vi "Grab Versions.vi"() -> (2 "Selection":string, 3 "Strings and Values":cluster{"string":string, "value":string}[](array[cluster]))   [LabVIEW 2021, in "TSC Button Editor.lvclass"]
doc: "See all of the available versions to save the button for compatiblity.\n\n<b>Code Developed By:</b>\nTechnology Service Corporation\n1983 S Liberty Drive\nBloomington, IN 47403\nwww.tsc.com/atcs\n\nDeveloper:\nDaniel Coons"
uses:
  TSC Button Editor.lvclass
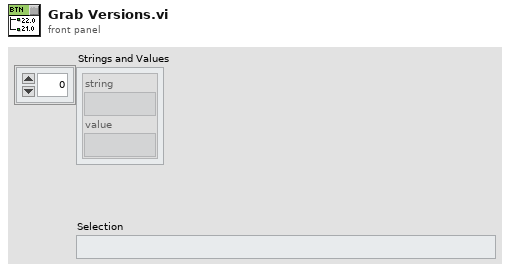
[diagram p1: front panel]
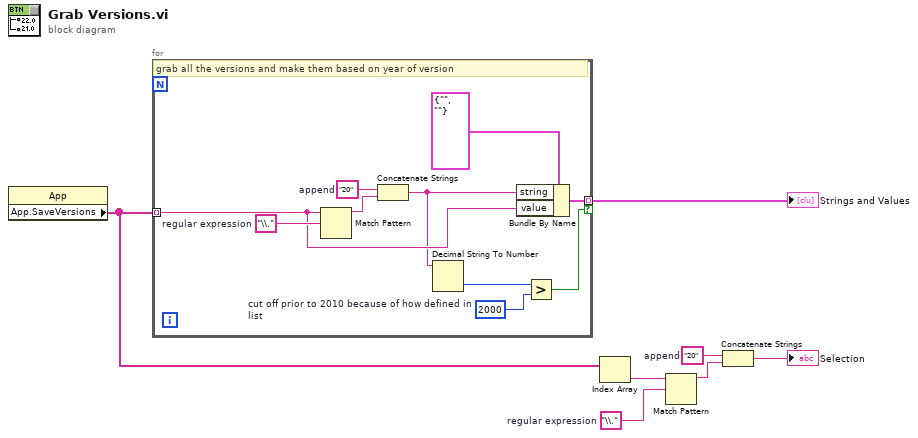
[diagram p0: block diagram]
diagram:
  w3 = "20"  # append
  w5 = "\\."  # regular expression
  n1 = property class="App"() -> ("App.SaveVersions"=w2:string[])  [unwired: 2 in, 2 out]
  n2 = for {
    tunnel: w2 -> [w13] mode=indexing
    tunnel: [w12] -> w1 mode=indexing if=w8
    w9 = 2000  # cut off prior to 2010 because of how defined in list
    w15 = "20"  # append
    w17 = "\\."  # regular expression
    # "grab all the versions and make them based on year of version"
    n3 = Match Pattern(string=w13, regular expression=w17) -> (before substring=w16:string)  [unwired: 1 in, 3 out]
    n4 = Concatenate Strings(w15, w16) -> (w11:string)
    n5 = Decimal String To Number(string=w11) -> (number=w10:i32)  [unwired: 2 in, 1 out]
    n6 = Bundle By Name(cluster=cluster{"string":string, "value":string} {"string"="", "value"=""}, "string"=w11, "value"=w13) -> (w12:cluster{"string":string, "value":string})
    n7 = Greater?(x=w10, y=w9) -> (0:w8:bool)
  }
  "Strings and Values" <- w1
  n8 = Index Array(array=w2) -> (element=w6:string)  [unwired: 1 in]
  n9 = Match Pattern(string=w6, regular expression=w5) -> (before substring=w4:string)  [unwired: 1 in, 3 out]
  n10 = Concatenate Strings(w3, w4) -> (→"Selection":string)
